vi "MotorCommand.vi"(2 "Parameter":i32, 3 "COM Port in":refnum<visa-resource-name>, 7 "Command":T1(ring), 9 "entrée d'erreur":errorcluster caption="error in (no error)") -> (0 "COM Port out":refnum<visa-resource-name>, 1 "Error Code":i32, 6 "error out":errorcluster)   [LabVIEW 2009]
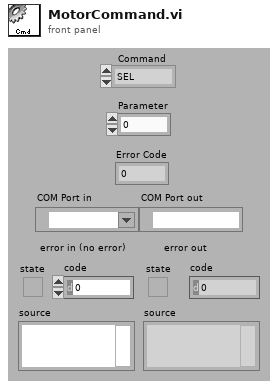
[diagram p1: front panel]
types:
  T1 = enum16{"SEL", "INIT", "MVT", "VMIN", "VMAX", "ACC", "POS", "MPAS", "INT", "JEU", "OFFSET", "L", "B", "STOP"}
  T2 = enum16{"?SEL", "?POS", "?VMIN", "?VMAX", "?ACC", "?MPAS", "?INT", "?JEU", "?OFFSET", "?L", "?FDC", "??", "?ST", "?MVT"}
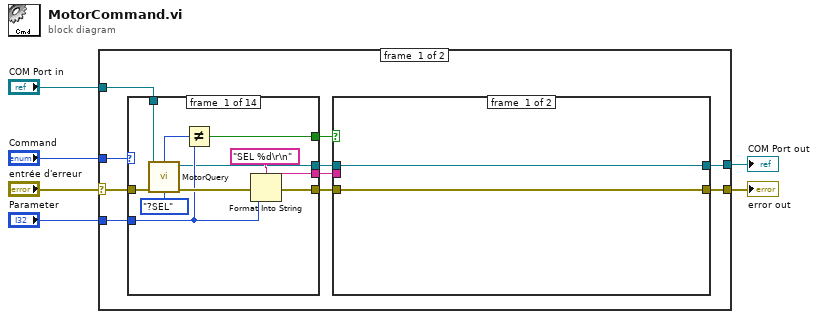
[diagram p0: block diagram]
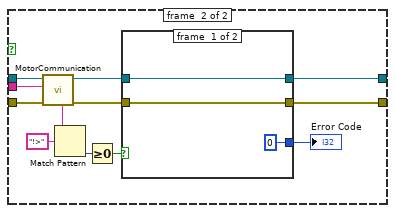
[diagram p2: hidden frame]
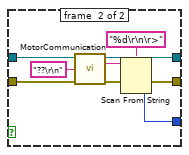
[diagram p3: hidden frame]
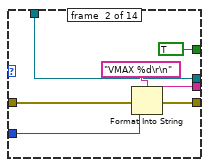
[diagram p4: hidden frame]
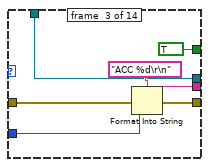
[diagram p5: hidden frame]
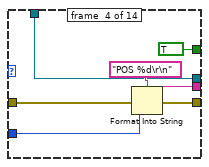
[diagram p6: hidden frame]
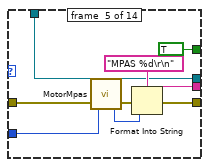
[diagram p7: hidden frame]
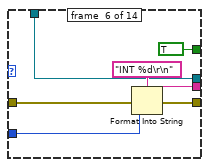
[diagram p8: hidden frame]
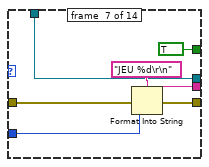
[diagram p9: hidden frame]
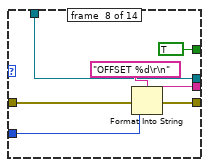
[diagram p10: hidden frame]
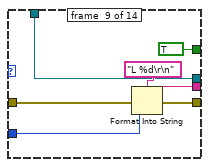
[diagram p11: hidden frame]
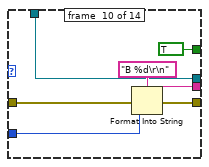
[diagram p12: hidden frame]
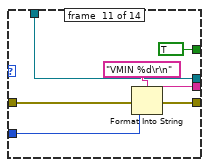
[diagram p13: hidden frame]
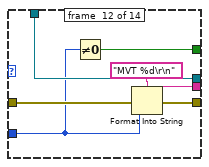
[diagram p14: hidden frame]
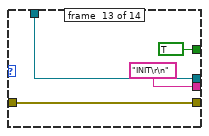
[diagram p15: hidden frame]
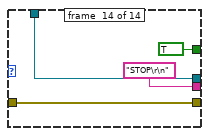
[diagram p16: hidden frame]
diagram:
  n1 = case shown="No Error" "entrée d'erreur" {
    selector: "entrée d'erreur" -> [w12 w142]
    tunnel: "Command" -> [w16 _]
    tunnel: "COM Port in" -> [w8 w141]
    tunnel: [w14 w142] -> w5
    tunnel: [w13 w141] -> w4
    tunnel: "Parameter" -> [w11 _]
    frame #0 {
      n2 = case shown="\"MVT\"" w16 {
        tunnel: w12 -> [w50 w60 w67 w74 w80 w90 w97 w104 w111 w118 w125 w132 w136 w140]
        tunnel: [w53 w59 w66 w73 w83 w89 w96 w103 w110 w117 w124 w131 w136 w140] -> w15
        tunnel: [w51 w57 w64 w71 w82 w87 w94 w101 w108 w115 w122 w129 "INIT\r\n" ("chaîne de format") "STOP\r\n" ("chaîne de format")] -> w10
        tunnel: w11 -> [w46 w56 w63 w69 w78 w86 w93 w100 w107 w114 w121 w127 _ _]
        tunnel: w8 -> [w47 w54 w61 w70 w75 w84 w91 w98 w105 w112 w119 w128 w133 w137]
        tunnel: [w44 TRUE TRUE TRUE TRUE TRUE TRUE TRUE TRUE TRUE TRUE w126 TRUE TRUE] -> w9
        tunnel: [w43 w54 w61 w70 w75 w84 w91 w98 w105 w112 w119 w128 w133 w137] -> w7
        frame #0 {
          n3 = call "MotorQuery.vi"("VISA in"=w47, "Command"=T2."?SEL", "entrée d'erreur"=w50) -> ("VISA out"=w43:refnum<visa-resource-name>, "I32 Result"=w45:i32, "sortie d'erreur"=w49:errorcluster)  [unwired: 4 out]
          n4 = Not Equal?(x=w45, y=w46) -> (x != y?=w44:bool)
          n5 = Format Into String(format string="SEL %d\r\n" ("chaîne de format"), error in=w49, w46) -> (resulting string=w51:string, error out=w53:errorcluster)  [unwired: 1 in]
        }
        frame #1 {
          n6 = Format Into String(format string="VMAX %d\r\n" ("chaîne de format"), error in=w60, w56) -> (resulting string=w57:string, error out=w59:errorcluster)  [unwired: 1 in]
        }
        frame #2 {
          n7 = Format Into String(format string="ACC %d\r\n" ("chaîne de format"), error in=w67, w63) -> (resulting string=w64:string, error out=w66:errorcluster)  [unwired: 1 in]
        }
        frame #3 {
          n8 = Format Into String(format string="POS %d\r\n" ("chaîne de format"), error in=w74, w69) -> (resulting string=w71:string, error out=w73:errorcluster)  [unwired: 1 in]
        }
        frame #4 {
          n9 = call "MotorMpas.vi"("entrée d'erreur 2"=w80, "Parameter"=w78) -> ("entrée d'erreur"=w79:errorcluster, "Numérique"=w77:i32)
          n10 = Format Into String(format string="MPAS %d\r\n" ("chaîne de format"), error in=w79, w77) -> (resulting string=w82:string, error out=w83:errorcluster)  [unwired: 1 in]
        }
        frame #5 {
          n11 = Format Into String(format string="INT %d\r\n" ("chaîne de format"), error in=w90, w86) -> (resulting string=w87:string, error out=w89:errorcluster)  [unwired: 1 in]
        }
        frame #6 {
          n12 = Format Into String(format string="JEU %d\r\n" ("chaîne de format"), error in=w97, w93) -> (resulting string=w94:string, error out=w96:errorcluster)  [unwired: 1 in]
        }
        frame #7 {
          n13 = Format Into String(format string="OFFSET %d\r\n" ("chaîne de format"), error in=w104, w100) -> (resulting string=w101:string, error out=w103:errorcluster)  [unwired: 1 in]
        }
        frame #8 {
          n14 = Format Into String(format string="L %d\r\n" ("chaîne de format"), error in=w111, w107) -> (resulting string=w108:string, error out=w110:errorcluster)  [unwired: 1 in]
        }
        frame #9 {
          n15 = Format Into String(format string="B %d\r\n" ("chaîne de format"), error in=w118, w114) -> (resulting string=w115:string, error out=w117:errorcluster)  [unwired: 1 in]
        }
        frame #10 {
          n16 = Format Into String(format string="VMIN %d\r\n" ("chaîne de format"), error in=w125, w121) -> (resulting string=w122:string, error out=w124:errorcluster)  [unwired: 1 in]
        }
        frame #11 {
          n17 = Not Equal To 0?(x=w127) -> (x != 0?=w126:bool)
          n18 = Format Into String(format string="MVT %d\r\n" ("chaîne de format"), error in=w132, w127) -> (resulting string=w129:string, error out=w131:errorcluster)  [unwired: 1 in]
        }
        frame #12 {
        }
        frame #13 {
        }
      }
      n19 = case shown="True" w9 {
        tunnel: w15 -> [w18 w24]
        tunnel: [w18 w27] -> w14
        tunnel: [w17 w26] -> w13
        tunnel: w10 -> [_ w23]
        tunnel: w7 -> [w17 w20]
        frame #0 {
        }
        frame #1 {
          n20 = call "MotorCommunication.vi"("Question"=w23, "error out"=w24, "COM Port in"=w20) -> ("error IO"=w19:errorcluster, "COM Port out"=w22:refnum<visa-resource-name>, "Answer"=w21:string)  [unwired: 4 out]
          n21 = Match Pattern(string=w21, regular expression="!>" ("expression")) -> (offset past match=w29:i32)  [unwired: 4 out]
          n22 = Greater Or Equal To 0?(x=w29) -> (x >= 0?=w28:bool)
          n23 = case shown="True" w28 {
            tunnel: w19 -> [w33 w35]
            tunnel: w22 -> [w32 w42]
            tunnel: [w33 w37] -> w27
            tunnel: [w32 w40] -> w26
            tunnel: [0 w36] -> w25
            frame #0 {
            }
            frame #1 {
              n24 = call "MotorCommunication.vi"("Question"="??\r\n" ("buffer à écrire"), "error out"=w35, "COM Port in"=w42) -> ("error IO"=w38:errorcluster, "COM Port out"=w40:refnum<visa-resource-name>, "Answer"=w34:string)  [unwired: 4 out]
              n25 = Scan From String(format string="%d\r\n\r>" ("chaîne de format"), input string=w34, error in=w38) -> (error out=w37:errorcluster, output 1=w36:i32)  [unwired: 1 in, 3 out]
            }
          }
          "Error Code" <- w25
        }
      }
    }
    frame #1 {
    }
  }
  "error out" <- w5
  "COM Port out" <- w4
